vi "ex_IncrementFilename.vi"(4 "name base":string) -> (1 "new name":string)   [LabVIEW 2017]
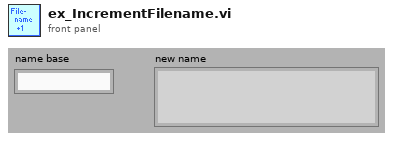
[diagram p1: front panel]
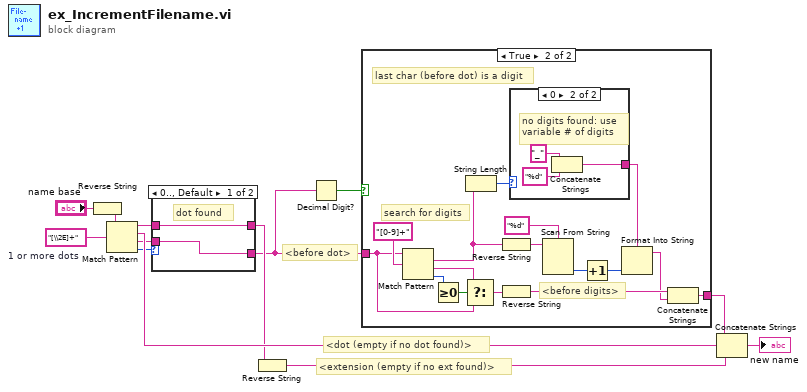
[diagram p0: block diagram]
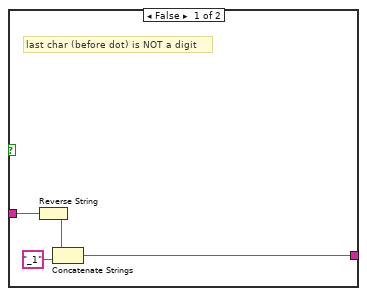
[diagram p2: hidden frame]
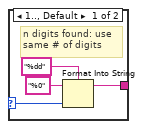
[diagram p3: hidden frame]
diagram:
  w12 = "[\\2E]+"  # 1 or more dots
  # "<dot (empty if no dot found)>"
  # "<before dot>"
  # "<extension (empty if no ext found)>"
  n1 = Reverse String(1:"name base") -> (0:w13:string)
  n2 = Match Pattern(string=w13, regular expression=w12) -> (before substring=w6:string, match substring=w9:string, after substring=w7:string, offset past match=w8:i32)  [unwired: 1 out]
  n3 = case shown="0.., Default" w8 {
    tunnel: w7 -> [w14 w16]
    tunnel: w6 -> [w15 w17]
    tunnel: [w14 w17] -> w2
    tunnel: [w15 w16] -> w3
    frame 0.., Default {
      # "dot found"
    }
    frame -1 {
      # "no dot found"
    }
  }
  n4 = Reverse String(1:w3) -> (0:w10:string)
  n5 = Decimal Digit?(1:w2) -> (0:w1:bool)
  n6 = case shown="True" w1 {
    tunnel: [w21 w37] -> w11
    tunnel: w2 -> [w20 w28]
    frame False {
      # "last char (before dot) is NOT a digit"
      n7 = Reverse String(1:w20) -> (0:w18:string)
      n8 = Concatenate Strings(w18, "_1" ("Substring")) -> (w21:string)
    }
    frame True {
      # "last char (before dot) is a digit"
      # "<before digits>"
      # "search for digits"
      n9 = Match Pattern(string=w28, regular expression="[0-9]+") -> (match substring=w34:string, after substring=w30:string, offset past match=w32:i32)  [unwired: 2 out]
      n10 = Greater Or Equal To 0?(x=w32) -> (x >= 0?=w31:bool)
      n11 = Select(t=w30, s=w31, f=w28) -> (s? t:f=w29:string)
      n12 = String Length(string=w34) -> (length=w24:i32)
      n13 = Reverse String(1:w34) -> (0:w27:string)
      n14 = Reverse String(1:w29) -> (0:w36:string)
      n15 = case shown="0" w24 {
        selector: w24 -> [w39 _]
        tunnel: [w41 w43] -> w23
        frame 1.., Default {
          # "n digits found: use\nsame # of digits"
          n16 = Format Into String(format string="%dd" ("Format String"), initial string="%0" ("Format String"), w39) -> (resulting string=w41:string)  [unwired: 1 in, 1 out]
        }
        frame 0 {
          # "no digits found: use\nvariable # of digits"
          n17 = Concatenate Strings("_" ("Substring"), "%d") -> (w43:string)
        }
      }
      n18 = Scan From String(format string="%d" ("Format String"), input string=w27) -> (output 1=w26:i32)  [unwired: 2 in, 4 out]
      n19 = Increment(x=w26) -> (x+1=w25:i32)
      n20 = Format Into String(format string=w23, w25) -> (resulting string=w33:string)  [unwired: 2 in, 1 out]
      n21 = Concatenate Strings(w36, w33) -> (w37:string)
    }
  }
  n22 = Concatenate Strings(w11, w9, w10) -> (→"new name":string)
